vi "Create TC Sections.vi"(8 "error in (no error)":errorcluster, 10 "Channel Data In":T3 {"Device Chan Total" max=32 step=1; "Thermocouple"."Temperature Units" items=["Celcius", "Fahrenheit", "Kelvin", "Rankine", "Volts"]; "Thermocouple"."Thermocouple Type" items=["J", "K", "T", "E", "N", "B", "R", "S", "Raw Voltage"]}, 11 "Device Configuration Data In in":T1 {"Current Section Ref" format="%.0x"; "simTC Section Refs" format="%.0x"; "Voltage Section Ref" format="%.0x"; "Custom Device Ref" format="%.0x"}) -> (0 "error out":errorcluster, 3 "Device Configuration Data In out":T1 {"Current Section Ref" format="%.0x"; "simTC Section Refs" format="%.0x"; "Voltage Section Ref" format="%.0x"; "Custom Device Ref" format="%.0x"})   [LabVIEW 2011, in "Simulated Thermocouple Custom Device.lvlib"]
uses:
  Simulated Thermocouple Custom Device.lvlib
  New Channel Data.ctl
  TC Selector.ctl
  TC Unit Selector.ctl
  Device Config data.ctl
  <vilib>/NI Veristand/Custom Device API/Custom Device Item Ref.ctl
  <vilib>/NI Veristand/Custom Device API/Custom Device Channel.ctl
  <vilib>/NI Veristand/Custom Device API/Custom Device Channel Type.ctl
  Calibration Config Data.ctl
  TC Section Config Data.ctl
  simTC Global GUIDs.vi
  <vilib>/NI Veristand/Custom Device API/Set Item Property (Variant).vi
  <vilib>/NI Veristand/Custom Device API/Custom Device API.lvlib
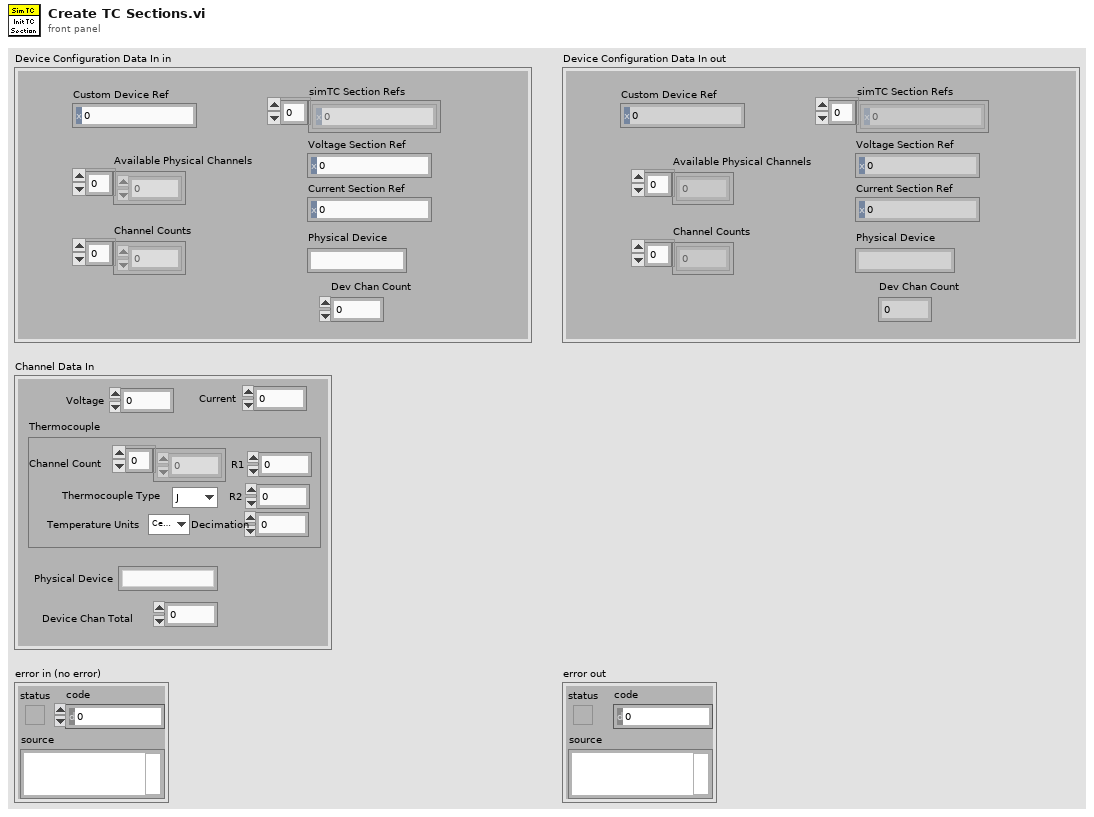
[diagram p1: front panel]
types:
  T1 = typedef "Simulated Thermocouple Custom Device.lvlib/Device Config data.ctl" = cluster{"Custom Device Ref":T2, "Voltage Section Ref":T2, "simTC Section Refs":T2[], "Current Section Ref":T2, "Physical Device":string, "Available Physical Channels":i32[], "Channel Counts":u32[], "Dev Chan Count":u32}
  T2 = typedef "Custom Device API.lvlib/Custom Device Item Ref.ctl" = u64
  T3 = typedef "Simulated Thermocouple Custom Device.lvlib/New Channel Data.ctl" = cluster{"Voltage":u32, "Current":u32, "Thermocouple":cluster{"R1":dbl, "R2":dbl, "Decimation":u32, "Thermocouple Type":T4, "Temperature Units":T5, "Channel Count":u32[]}, "Physical Device":string, "Device Chan Total":u32}
  T4 = typedef "Simulated Thermocouple Custom Device.lvlib/TC Selector.ctl" = u16
  T5 = typedef "Simulated Thermocouple Custom Device.lvlib/TC Unit Selector.ctl" = u16
  T6 = typedef "Simulated Thermocouple Custom Device.lvlib/TC Section Config Data.ctl" = cluster{"Temperature Units":T5, "Thermocouple Type":T4}
  T7 = typedef "Simulated Thermocouple Custom Device.lvlib/Calibration Config Data.ctl" = cluster{"Local SimTC Chan":string, "Samples To Collect":dbl, "Cal Channel TC Type":T4, "Cal Step Settling Time":dbl}
  T8 = typedef "Custom Device API.lvlib/Custom Device Channel.ctl" = cluster{"Type":T9, "Units":string, "Default Value":dbl, "Faultable":bool, "Scalable":bool}
  T9 = typedef "Custom Device API.lvlib/Custom Device Channel Type.ctl" = enum16{"Input", "Output"}
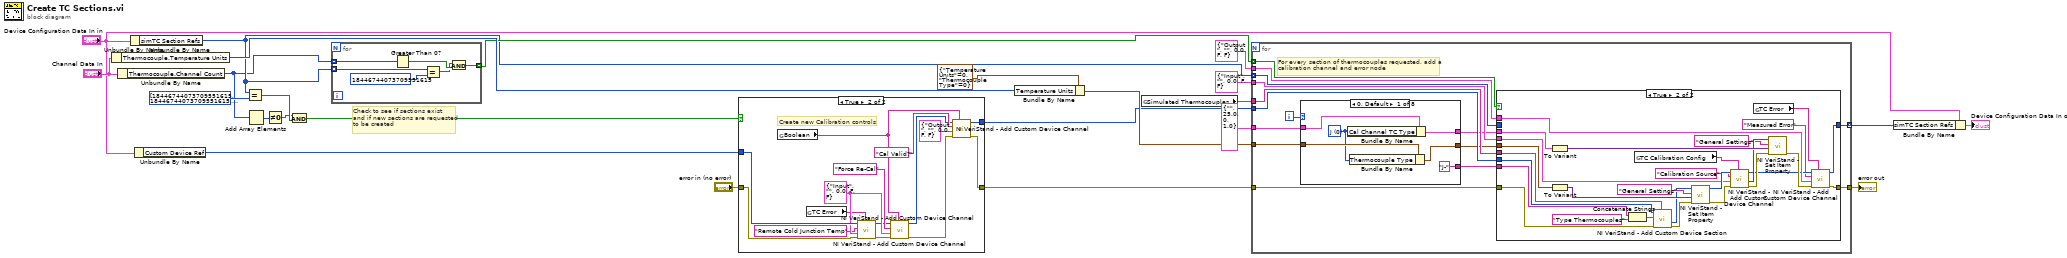
[diagram p0: block diagram]
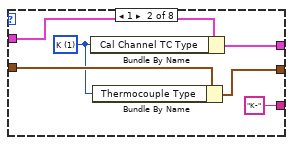
[diagram p2: hidden frame]
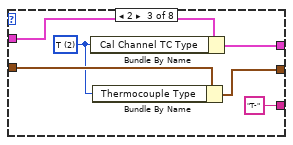
[diagram p3: hidden frame]
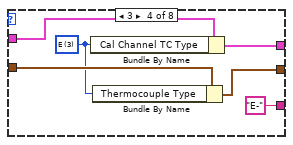
[diagram p4: hidden frame]
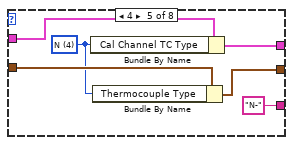
[diagram p5: hidden frame]
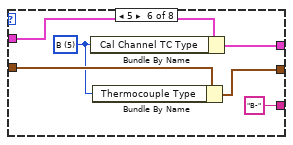
[diagram p6: hidden frame]
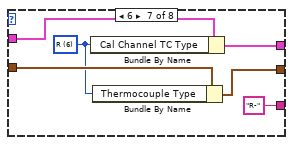
[diagram p7: hidden frame]
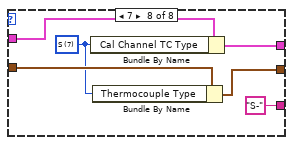
[diagram p8: hidden frame]
diagram:
  # "Check to see if sections exist\nand if new sections are requested\nto be created"
  n1 = Unbundle By Name("Channel Data In") -> ("Thermocouple.Temperature Units"=w12:T5)
  n2 = Unbundle By Name("Channel Data In") -> ("Thermocouple.Channel Count"=w6:u32[])
  n3 = Unbundle By Name("Device Configuration Data In in") -> ("simTC Section Refs"=w8:T2[])
  n4 = Unbundle By Name("Device Configuration Data In in") -> ("Custom Device Ref"=w1:T2)
  n5 = Equal?(x=w8, y=T2[] [18446744073709551615, 18446744073709551615, 18446744073709551615, 18446744073709551615, 18446744073709551615, 18446744073709551615, 18446744073709551615, 18446744073709551615]) -> (x = y?=w5:bool)
  n6 = Add Array Elements(numeric array=w6) -> (sum=w3:u32)
  n7 = Not Equal To 0?(x=w3) -> (x != 0?=w2:bool)
  n8 = And(x=w2, y=w5) -> (x .and. y?=w4:bool)
  n9 = for {
    tunnel: w8 -> [w30] mode=indexing
    tunnel: w6 -> [w29] mode=indexing
    tunnel: [w28] -> w9 mode=indexing
    n10 = Greater Than 0?(x=w29) -> (x > 0?=w27:bool)
    n11 = Equal?(x=w30, y=T2 18446744073709551615) -> (x = y?=w26:bool)
    n12 = And(x=w26, y=w27) -> (x .and. y?=w28:bool)
  }
  n13 = case shown="True" w4 {
    tunnel: w1 -> [w31 w47]
    tunnel: "error in (no error)" -> [w32 w44]
    tunnel: [w32 w39] -> w14
    tunnel: [w31 w33] -> w15
    frame False {
    }
    frame True {
      w46 = T8 {"Type"=enum."Input", "Units"="", "Default Value"=0.0, "Faultable"=FALSE, "Scalable"=FALSE} ("Channel")
      # "Create new Calibration controls"
      n14 = global read "simTC Global GUIDs.vi" "Boolean"() -> (w36:string)
      n15 = global read "simTC Global GUIDs.vi" "TC Error"() -> (w35:string)
      n16 = call <vilib>:"NI VeriStand - Add Custom Device Channel.vi"("GUID (Default Channel)"=w35, "error in (no error)"=w44, "Channel"=w46, "Channel Name"="Remote Cold Junction Temp", "Parent Ref in"=w47) -> ("error out"=w45:errorcluster, "Parent Ref out"=w41:T2)  [unwired: 3 in, 2 out]
      n17 = call <vilib>:"NI VeriStand - Add Custom Device Channel.vi"("GUID (Default Channel)"=w36, "error in (no error)"=w45, "Channel"=w46, "Channel Name"="Force Re-Cal", "Parent Ref in"=w41) -> ("error out"=w43:errorcluster, "Parent Ref out"=w37:T2)  [unwired: 3 in, 2 out]
      n18 = call <vilib>:"NI VeriStand - Add Custom Device Channel.vi"("GUID (Default Channel)"=w36, "error in (no error)"=w43, "Channel"=T8 {"Type"=enum."Output", "Units"="", "Default Value"=0.0, "Faultable"=FALSE, "Scalable"=FALSE}, "Channel Name"="Cal Valid?", "Parent Ref in"=w37) -> ("error out"=w39:errorcluster, "Parent Ref out"=w33:T2)  [unwired: 3 in, 2 out]
    }
  }
  n19 = Bundle By Name(cluster=T6 {"Temperature Units"=0, "Thermocouple Type"=0} ("TC Section Config Data"), "Temperature Units"=w12) -> (w19:T6)
  n20 = global read "simTC Global GUIDs.vi" "Simulated Thermocouples"() -> (w17:string)
  n21 = for {
    tunnel: T7 {"Local SimTC Chan"="", "Samples To Collect"=25.0, "Cal Channel TC Type"=0, "Cal Step Settling Time"=1.0} ("Cal Info") -> [w52]
    tunnel: T8 {"Type"=enum."Output", "Units"="", "Default Value"=0.0, "Faultable"=FALSE, "Scalable"=FALSE} ("Channel") -> [w62]
    tunnel: T8 {"Type"=enum."Input", "Units"="", "Default Value"=0.0, "Faultable"=FALSE, "Scalable"=FALSE} ("Channel") -> [w61]
    tunnel: w19 -> [w51]
    tunnel: [w60] -> w18
    tunnel: w17 -> [w59]
    tunnel: w15 -> [w58]
    tunnel: w14 -> [w57]
    tunnel: w9 -> [w56] mode=indexing
    tunnel: [w53] -> w10 mode=indexing
    tunnel: w8 -> [w49] mode=indexing
    i -> [w55]
    # "For every section of thermocouples requested, add a\ncalibration channel and error node"
    n22 = case shown="0, Default" w55 {
      tunnel: ["J-" "K-" "T-" "E-" "N-" "B-" "R-" "S-"] -> w54
      tunnel: w52 -> [w67 w73 w79 w85 w90 w96 w103 w109]
      tunnel: [w66 w72 w78 w84 w91 w97 w102 w108] -> w48
      tunnel: w51 -> [w65 w70 w77 w83 w89 w95 w100 w107]
      tunnel: [w63 w71 w76 w82 w88 w94 w101 w106] -> w50
      frame 0, Default {
        w64 = T4 0 items=["J", "K", "T", "E", "N", "B", "R", "S"] ("Cal Channel TC Type")
        n23 = Bundle By Name(cluster=w67, "Cal Channel TC Type"=w64) -> (w66:T7)
        n24 = Bundle By Name(cluster=w65, "Thermocouple Type"=w64) -> (w63:T6)
      }
      frame 1 {
        w69 = T4 1 items=["J", "K", "T", "E", "N", "B", "R", "S"] ("Cal Channel TC Type")
        n25 = Bundle By Name(cluster=w73, "Cal Channel TC Type"=w69) -> (w72:T7)
        n26 = Bundle By Name(cluster=w70, "Thermocouple Type"=w69) -> (w71:T6)
      }
      frame 2 {
        w75 = T4 2 items=["J", "K", "T", "E", "N", "B", "R", "S"] ("Cal Channel TC Type")
        n27 = Bundle By Name(cluster=w79, "Cal Channel TC Type"=w75) -> (w78:T7)
        n28 = Bundle By Name(cluster=w77, "Thermocouple Type"=w75) -> (w76:T6)
      }
      frame 3 {
        w81 = T4 3 items=["J", "K", "T", "E", "N", "B", "R", "S"] ("Cal Channel TC Type")
        n29 = Bundle By Name(cluster=w85, "Cal Channel TC Type"=w81) -> (w84:T7)
        n30 = Bundle By Name(cluster=w83, "Thermocouple Type"=w81) -> (w82:T6)
      }
      frame 4 {
        w87 = T4 4 items=["J", "K", "T", "E", "N", "B", "R", "S"] ("Cal Channel TC Type")
        n31 = Bundle By Name(cluster=w90, "Cal Channel TC Type"=w87) -> (w91:T7)
        n32 = Bundle By Name(cluster=w89, "Thermocouple Type"=w87) -> (w88:T6)
      }
      frame 5 {
        w93 = T4 5 items=["J", "K", "T", "E", "N", "B", "R", "S"] ("Cal Channel TC Type")
        n33 = Bundle By Name(cluster=w96, "Cal Channel TC Type"=w93) -> (w97:T7)
        n34 = Bundle By Name(cluster=w95, "Thermocouple Type"=w93) -> (w94:T6)
      }
      frame 6 {
        w99 = T4 6 items=["J", "K", "T", "E", "N", "B", "R", "S"] ("Cal Channel TC Type")
        n35 = Bundle By Name(cluster=w103, "Cal Channel TC Type"=w99) -> (w102:T7)
        n36 = Bundle By Name(cluster=w100, "Thermocouple Type"=w99) -> (w101:T6)
      }
      frame 7 {
        w105 = T4 7 items=["J", "K", "T", "E", "N", "B", "R", "S"] ("Cal Channel TC Type")
        n37 = Bundle By Name(cluster=w109, "Cal Channel TC Type"=w105) -> (w108:T7)
        n38 = Bundle By Name(cluster=w107, "Thermocouple Type"=w105) -> (w106:T6)
      }
    }
    n39 = case shown="True" w56 {
      tunnel: w58 -> [_ w140]
      tunnel: w59 -> [_ w139]
      tunnel: w57 -> [w112 w138]
      tunnel: [w112 w121] -> w60
      tunnel: w50 -> [_ w134]
      tunnel: w61 -> [_ w124]
      tunnel: w62 -> [_ w125]
      tunnel: w48 -> [_ w129]
      tunnel: w54 -> [_ w114]
      tunnel: [w111 w113] -> w53
      tunnel: w49 -> [w111 _]
      frame False {
      }
      frame True {
        n40 = To Variant(anything=w129) -> (Variant=w130:variant)
        n41 = To Variant(anything=w134) -> (Variant=w136:variant)
        n42 = Concatenate Strings(w114, "Type Thermocouples" ("Section Name")) -> (w116:string)
        n43 = global read "simTC Global GUIDs.vi" "TC Calibration Config"() -> (w120:string)
        n44 = call <vilib>:"NI VeriStand - Add Custom Device Section.vi"("GUID (Default Section)"=w139, "error in (no error)"=w138, "Section Name"=w116, "Parent Ref in"=w140) -> ("error out"=w137:errorcluster, "Section Ptr"=w133:T2)  [unwired: 4 in, 2 out]
        n45 = call-poly <vilib>:"NI VeriStand - Set Item Property.vi"("error in (no error)"=w137, "Value"=w136, "Property Name"="General Settings", "Item Ref in"=w133) -> ("error out"=w132:errorcluster, "Item Ref out"=w131:T2)  [unwired: 5 in, 1 out]
        n46 = call <vilib>:"NI VeriStand - Add Custom Device Channel.vi"("GUID (Default Channel)"=w120, "error in (no error)"=w132, "Channel"=w124, "Channel Name"="Calibration Source", "Parent Ref in"=w131) -> ("error out"=w127:errorcluster, "Channel Ref"=w128:T2, "Parent Ref out"=w122:T2)  [unwired: 3 in, 1 out]
        n47 = global read "simTC Global GUIDs.vi" "TC Error"() -> (w117:string)
        n48 = call-poly <vilib>:"NI VeriStand - Set Item Property.vi"("error in (no error)"=w127, "Value"=w130, "Property Name"="General Settings", "Item Ref in"=w128) -> ("error out"=w123:errorcluster)  [unwired: 5 in, 2 out]
        n49 = call <vilib>:"NI VeriStand - Add Custom Device Channel.vi"("GUID (Default Channel)"=w117, "error in (no error)"=w123, "Channel"=w125, "Channel Name"="Measured Error", "Parent Ref in"=w122) -> ("error out"=w121:errorcluster, "Parent Ref out"=w113:T2)  [unwired: 3 in, 2 out]
      }
    }
  }
  "error out" <- w18
  n50 = Bundle By Name(cluster="Device Configuration Data In in", "simTC Section Refs"=w10) -> (→"Device Configuration Data In out":T1)
